vi "GetAllEquipmentAssets.vi"(8 "error in (no error)":errorcluster, 11 "service":refnum<class "IcmMessageService.lvclass">) -> (0 "error out":errorcluster, 3 "AssetNodes":T1[](array[typedef]))   [LabVIEW 2016]
doc: "Queries for all equipment asset nodes, which means they have operating states."
uses:
  <vilib>/addons/InsightCM/MessageBus/MessageService/IcmMessageService.lvclass
  <vilib>/addons/InsightCM/MessageBus/Base/controls/AssetState.ctl
  <vilib>/addons/InsightCM/MessageBus/Base/controls/KeyValuePair.ctl
  <vilib>/addons/InsightCM/MessageBus/Base/controls/Metric.ctl
  <vilib>/addons/InsightCM/MessageBus/Base/controls/AssetNodeReference.ctl
  <vilib>/addons/InsightCM/MessageBus/Base/controls/AssetNodeView.ctl
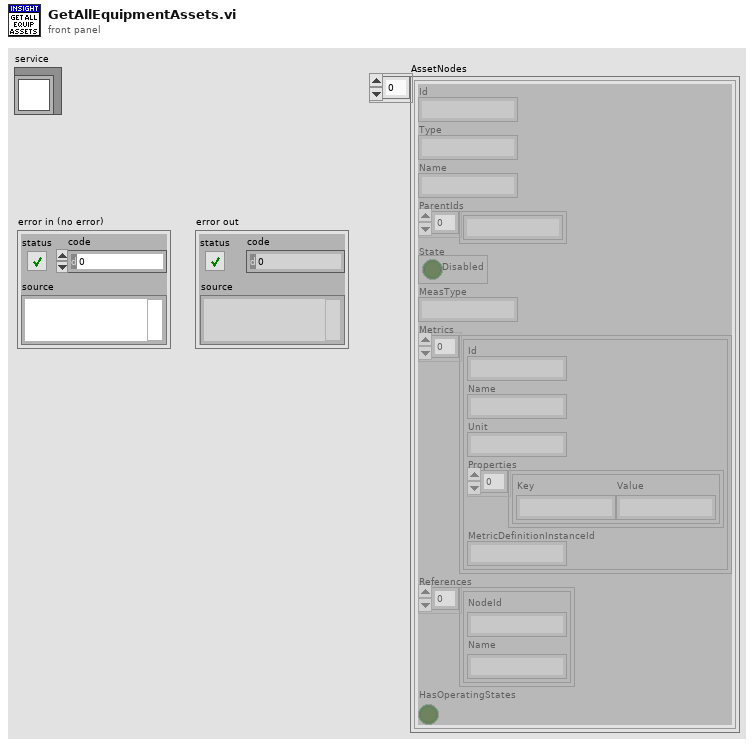
[diagram p1: front panel]
types:
  T1 = typedef "AssetNodeView.ctl" = cluster{"Id":string, "Type":string, "Name":string, "ParentIds":string[], "State":T2, "MeasType":string, "Metrics":T3[], "References":T5[], "HasOperatingStates":bool}
  T2 = typedef "AssetState.ctl" = cluster{"Disabled":bool}
  T3 = typedef "Metric.ctl" = cluster{"Id":string, "Name":string, "Unit":string, "Properties":T4[], "MetricDefinitionInstanceId":string}
  T4 = typedef "KeyValuePair.ctl" = cluster{"Key":string, "Value":string}
  T5 = typedef "AssetNodeReference.ctl" = cluster{"NodeId":string, "Name":string}
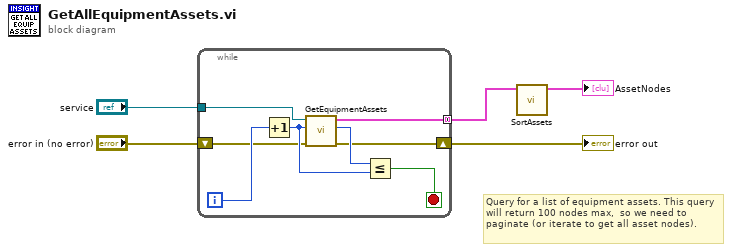
[diagram p0: block diagram]
diagram:
  # "Query for a list of equipment assets. This query will return 100 nodes max,  so we need to paginate (or iterate to get all asset nodes)."
  n1 = while {
    tunnel: [w9] -> w1 mode=concatenating
    shift-right: [w7] -> w4
    shift-left: "error in (no error)" -> [w8]
    tunnel: "service" -> [w6]
    i -> [w13]
    stop <- w10 stop-if-true
    n2 = Increment(x=w13) -> (x+1=w11:i32)
    n3 = call "GetEquipmentAssets.vi"("error in (no error)"=w8, "page"=w11, "service"=w6) -> ("error out"=w7:errorcluster, "pages"=w12:i32, "AssetNodes"=w9:T1[])  [unwired: 6 in]
    n4 = Less Or Equal?(x=w12, y=w11) -> (x <= y?=w10:bool)
  }
  "error out" <- w4
  n5 = call "SortAssets.vi"("AssetNodes in"=w1) -> ("AssetNodes out"=→"AssetNodes":T1[])  [unwired: 10 in]
